vi "IsValidVariable.vi"(4 "Value String in":string) -> (0 "IsVariable":bool, 2 "Variable Name":string)   [LabVIEW 2016]
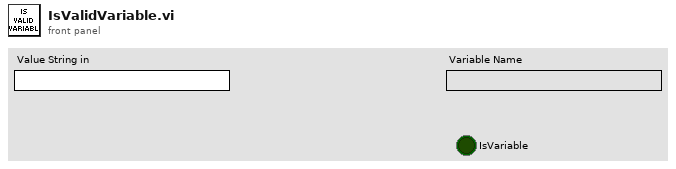
[diagram p1: front panel]
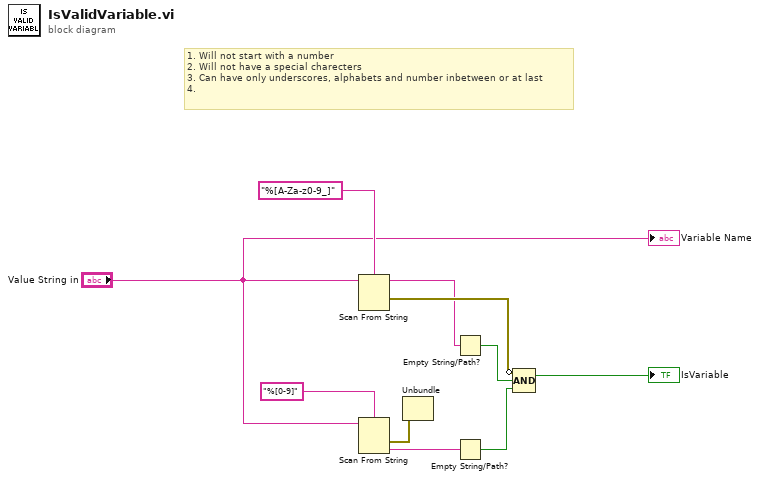
[diagram p0: block diagram]
diagram:
  # "1. Will not start with a number\n2. Will not have a special charecters\n3. Can have only underscores, alphabets and number inbetween or at last\n4."
  n1 = Scan From String(format string="%[A-Za-z0-9_]", input string="Value String in") -> (remaining string=w8:string, error out=w9:errorcluster)  [unwired: 4 in, 1 out]
  n2 = Scan From String(format string="%[0-9]", input string="Value String in") -> (error out=w6:errorcluster, output 1=w4:string)  [unwired: 3 in, 2 out]
  n3 = Unbundle(w6) -> ()  [unwired: 3 out]
  n4 = Empty String/Path?(string/path=w8) -> (empty?=w7:bool)
  n5 = Empty String/Path?(string/path=w4) -> (empty?=w2:bool)
  n6 = Compound Arithmetic op=AND(invert w9, w7, w2) -> (→"IsVariable":bool)
  "Variable Name" <- "Value String in"
